vi "Prepare WebSocket Upgrade Response.vi"(11 "Request":refnum<class "Request.lvclass">) -> (3 "WebSocket Response":refnum<class "WebSocketUpgradeResponse.lvclass">)   [LabVIEW 2020, in "Stream-Websocket.lvlib"]
uses:
  Stream-Websocket.lvlib
  lv-http-util/HTTP Utils/Request/Request.lvclass
  WebSocketUpgradeResponse/WebSocketUpgradeResponse.lvclass
  lv-http-util/HTTP Utils/Response/Response.lvclass
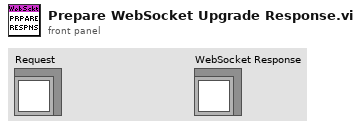
[diagram p1: front panel]
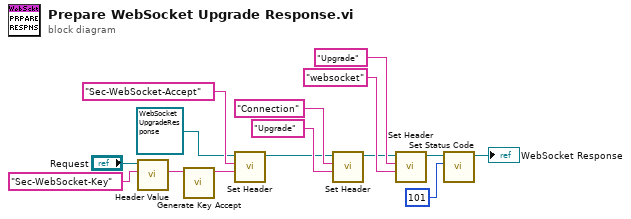
[diagram p0: block diagram]
diagram:
  n1 = call "Header Value.vi"("Header"="Sec-WebSocket-Key", "Request in"="Request") -> ("Value"=w13:string)  [unwired: 6 in, 3 out]
  n2 = call "Generate Key Accept.vi"("Sec-WebSocket-Key"=w13) -> ("Sec-WebSocket-Accept"=w2:string)  [unwired: 10 in]
  n3 = call "Set Header.vi"("Value"=w2, "Header"="Sec-WebSocket-Accept", "Response in"=refnum<class "WebSocketUpgradeResponse.lvclass"> refnum ("Stream-Websocket.lvlib:WebSocketUpgradeResponse.lvclass")) -> ("Response out"=w3:refnum<class "WebSocketUpgradeResponse.lvclass">)  [unwired: 6 in, 2 out]
  n4 = call "Set Header.vi"("Value"="Upgrade" ("Header"), "Header"="Connection", "Response in"=w3) -> ("Response out"=w5:refnum<class "WebSocketUpgradeResponse.lvclass">)  [unwired: 6 in, 2 out]
  n5 = call "Set Header.vi"("Value"="websocket" ("Header"), "Header"="Upgrade", "Response in"=w5) -> ("Response out"=w10:refnum<class "WebSocketUpgradeResponse.lvclass">)  [unwired: 6 in, 2 out]
  n6 = call "Set Status Code.vi"("Status Code"=u16 101, "Response in"=w10) -> ("Response out"=→"WebSocket Response":refnum<class "WebSocketUpgradeResponse.lvclass">)  [unwired: 8 in, 1 out]
